vi "log.vi"(6 "Operation Mode":enum16{"열기", "쓰기", "닫기"}(ring), 7 "error in (no error)":errorcluster caption="에러 입력(에러 없음)", 9 "System Log":string, 10 "Log Files":path) -> (0 "error out":errorcluster caption="에러 출력")   [LabVIEW 2014]
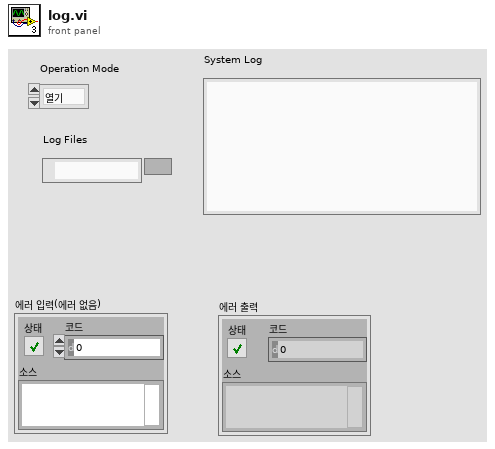
[diagram p1: front panel]
types:
  T1 = enum16{"open", "replace", "create", "open or create", "replace or create", "replace or create with confirmation"}
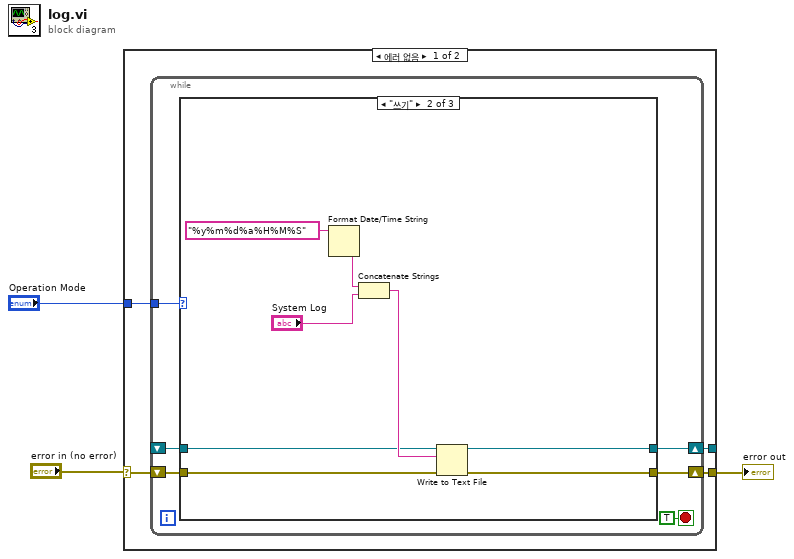
[diagram p0: block diagram]
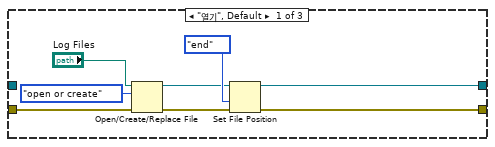
[diagram p2: hidden frame]
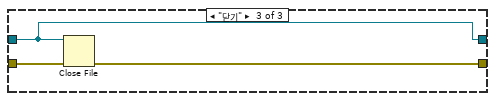
[diagram p3: hidden frame]
diagram:
  n1 = case shown="에러 없음" "error in (no error)" {
    selector: "error in (no error)" -> [w6 w33]
    tunnel: "Operation Mode" -> [w7 _]
    tunnel: [w5 _] -> _
    tunnel: [w4 w33] -> w1
    frame No Error {
      n2 = while {
        tunnel: w7 -> [w13]
        shift-right: [w10] -> w4
        shift-left: w6 -> [w12]
        shift-right: [w11] -> w5
        shift-left: _ -> [w9]
        stop <- TRUE stop-if-true
        n3 = case shown="\"쓰기\"" w13 {
          tunnel: w12 -> [w21 w29 w32]
          tunnel: [w16 w24 w30] -> w11
          tunnel: [w15 w23 w31] -> w10
          tunnel: w9 -> [_ w22 w30]
          frame "열기", Default {
            n4 = Open/Create/Replace File(file path (use dialog)="Log Files", error in=w21, operation (0:open)=T1."open or create" ("동작(0:open)")) -> (refnum out=w18:refnum<file>, error out=w17:errorcluster)  [unwired: 3 in, 1 out]
            n5 = Set File Position(refnum=w18, from (0:start)=enum16{"start", "end", "current"}."end" ("시작(0:시작)"), error in=w17) -> (refnum out=w16:refnum<file>, error out=w15:errorcluster)  [unwired: 1 in]
          }
          frame "쓰기" {
            n6 = Format Date/Time String(time format string (%c)="%y%m%d%a%H%M%S" ("시간 포맷 문자열 (%c)")) -> (date/time string=w27:string)  [unwired: 2 in]
            n7 = Concatenate Strings(w27, "System Log") -> (w25:string)
            n8 = Write to Text File(file (use dialog)=w22, text=w25, error in=w29) -> (refnum out=w24:refnum<file>, error out=w23:errorcluster)  [unwired: 1 in, 1 out]
          }
          frame "닫기" {
            n9 = Close File(refnum=w30, error in=w32) -> (error out=w31:errorcluster)  [unwired: 1 out]
          }
        }
      }
    }
    frame Error {
    }
  }
  "error out" <- w1
